vi "subGeneratePackets2.vi"(0 "Samples per Symbol":i32, 1 "Packet Pad \n[samples]":i32, 3 "PSK system parameters":T2, 5 "Tx IQ Sampling\nRate [s/sec]":dbl, 9 "Pulse Shaping Filter Parameters":T3, 11 "PN sequence order\nfor Sync Bits":i32, 12 "Packet Parameters":T1, 14 "Message Type":bool, 15 "path to JPEG file":path) -> (4 "Number of Packets":i32, 6 "Packets":cluster{"t0":dbl, "dt":dbl, "Y":cdb[]}[](array[cluster]), 10 "Symbol Rate":dbl, 13 "Transmitted picture":picture)   [LabVIEW 2019]
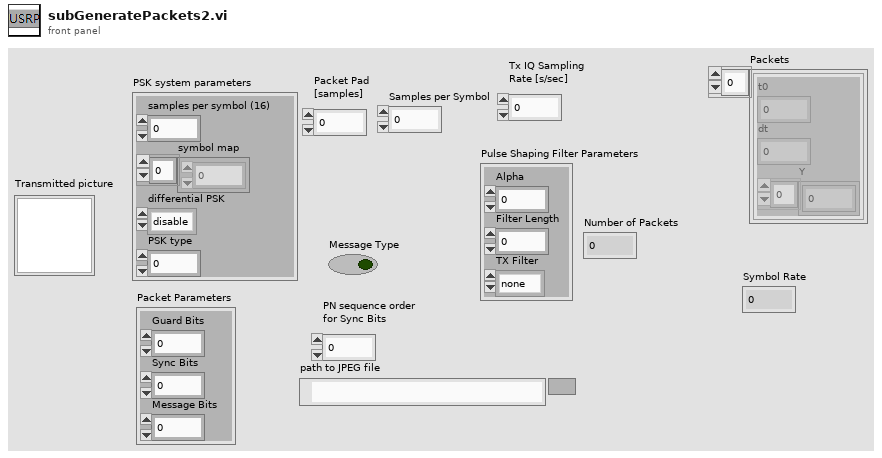
[diagram p1: front panel]
types:
  T1 = cluster{"Guard Bits ":i32, "Sync Bits":i32, "Message Bits":i32}
  T2 = cluster{"samples per symbol (16)":i32, "symbol map":cdb[], "differential PSK":enum16{"disable", "enable"}, "PSK type":u16}
  T3 = cluster{"Alpha":dbl, "Filter Length":i32, "TX Filter":enum16{"none", "Raised Cosine", "Root Raised Cos", "Gaussian"}}
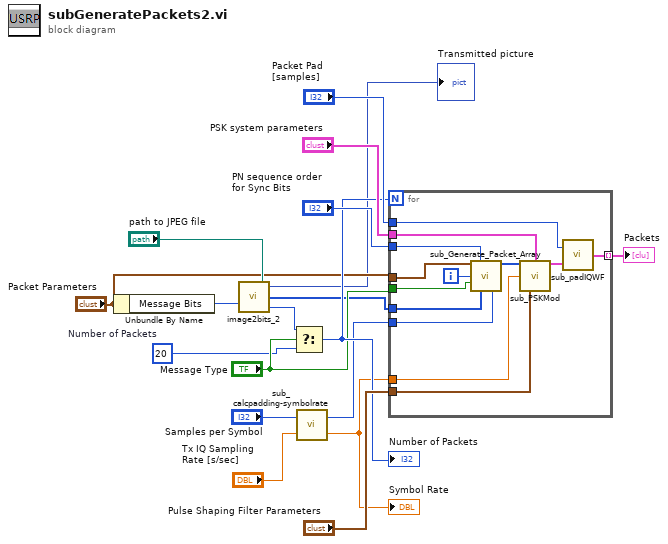
[diagram p0: block diagram]
diagram:
  w12 = 20  # Number of Packets
  n1 = Unbundle By Name("Packet Parameters") -> ("Message Bits"=w4:i32)
  n2 = call "image2bits_2.vi"("Packet\nMessage Length (bits)"=w4, "path to JPEG file"="path to JPEG file") -> ("Number of Packets"=w3:i32, "Bitstream with Guard"=w1:u8[], "Transmitted picture"=→"Transmitted picture":picture)  [unwired: 1 in]
  n3 = Select(t=w3, s="Message Type", f=w12) -> (s? t:f=w14:i32)
  "Number of Packets" <- w14
  n4 = call "sub_calcpadding-symbolrate.vi"("Tx IQ Sampling\nRate [s/sec]"="Tx IQ Sampling\nRate [s/sec]", "Samples per Symbol"="Samples per Symbol") -> ("Symbol Rate"=w8:dbl, "Padding Bits"=w10:i32)
  "Symbol Rate" <- w8
  n5 = for {
    N: w14 -> [_]
    tunnel: "Packet Parameters" -> [w28]
    tunnel: [w21] -> w11 mode=indexing
    tunnel: "Message Type" -> [w30]
    tunnel: w1 -> [w29]
    tunnel: "PN sequence order\nfor Sync Bits" -> [w27]
    tunnel: w10 -> [w26]
    tunnel: "PSK system parameters" -> [w24]
    tunnel: w8 -> [w23]
    tunnel: "Pulse Shaping Filter Parameters" -> [w22]
    tunnel: "Packet Pad \n[samples]" -> [w19]
    i -> [w31]
    n6 = call "sub_Generate_Packet_Array.vi"("Packet Parameters"=w28, "PN sequence order\nfor Sync"=w27, "Packet Number"=w31, "User defined bitstream?"=w30, "user  bitstream"=w29, "Cyclic Padding Bits"=w26) -> ("Output Packet"=w25:i8[])  [unwired: 9 in]
    n7 = call "sub_PSKMod.vi"("Packet to Transmit"=w25, "PSK system parameters"=w24, "Symbol Rate, Hz"=w23, "filter parameters"=w22) -> ("output complex waveform"=w20:cluster{"t0":dbl, "dt":dbl, "Y":cdb[]})  [unwired: 9 in, 2 out]
    n8 = call "sub_padIQWF.vi"("input complex waveform"=w20, "Packet Pad \n[samples]"=w19) -> ("output complex waveform"=w21:cluster{"t0":dbl, "dt":dbl, "Y":cdb[]})
  }
  "Packets" <- w11
